vi "FlatToRichhwval_BoolRequest.vi"(5 "OutputClusterType":T1, 11 "InputCluster":T2) -> (3 "OutputCluster":T1)   [LabVIEW 2025, in "Automotive-Vision-OOBService_server.lvlib"]
uses:
  Automotive-Vision-OOBService_server.lvlib
  hwval_BoolRequest_Flat.ctl
  hwval_BoolRequest.ctl
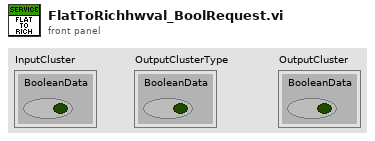
[diagram p1: front panel]
types:
  T1 = typedef "Automotive-Vision-OOBService_server.lvlib/hwval_BoolRequest.ctl" = cluster{"BooleanData":bool}
  T2 = typedef "Automotive-Vision-OOBService_server.lvlib/hwval_BoolRequest_Flat.ctl" = cluster{"BooleanData":bool}
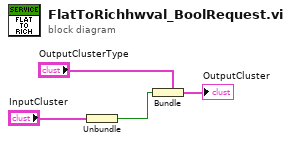
[diagram p0: block diagram]
diagram:
  n1 = Unbundle "Unbundle"("InputCluster") -> ("BooleanData"=w1:bool)
  n2 = Bundle "Bundle"(cluster="OutputClusterType", "BooleanData"=w1) -> (→"OutputCluster":T1)
